vi "Report Driver.vi"(4 "Both XL & PDF":bool, 6 "PDF":bool, 8 "error in":errorcluster, 10 "2D Data":string[][](array[string]), 11 "Header Data":string[](array[string])) -> (0 "error out":errorcluster, 3 "Pathout":path)   [LabVIEW 2017]
uses:
  controls/Excel.ctl
  controls/read.write.ctl
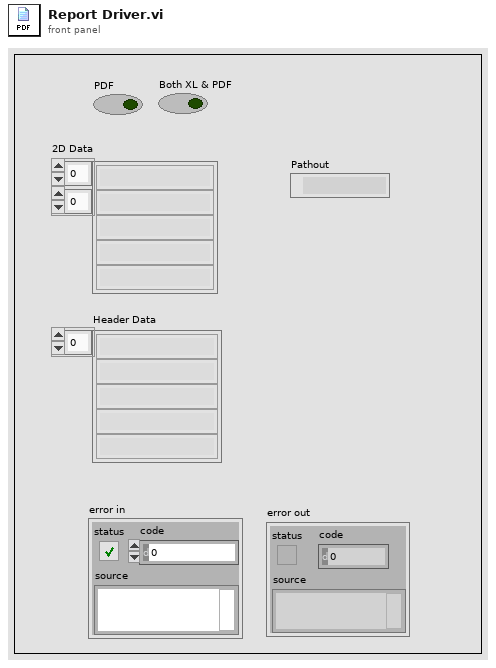
[diagram p1: front panel]
types:
  T1 = typedef "Excel.ctl" = enum16{"Open XL", "Create Hyperlink within Sheet", "Create Hyperlink between Sheets", "Hyperlink Folders", "Read Sheet names", "Print", "Print Preview", "print", "Open WB", "Copy Sheets", "Copy sheet to sheet", "Add Sheets", "Select Sheet", "Paste CLPBRD", "Read 1 Cell", "Read 2D", "Write 1 Cell", "Write 1 Cell No", "Write 2D String", "Write 2D Double", "Write 1D String", "Write 1D Double", "Merge Cells", "Borders", "Save", "Save As PDF", "Get Last Row Column Number", "Close Sheet", "Delete Sheet", "Close WB", "Close XL"}
  T2 = typedef "read.write.ctl" = cluster{"Cell Range":string, "Data 2D":string[][], "Select Sheet":string, "1 Data":string, "Data 1D":string[], "Font col":u32, "Bold":bool, "Font Size":i32, "Inside lines":bool}
  T3 = cluster{"Excel WB Path":path, "Read Only?":bool, "Password":string}
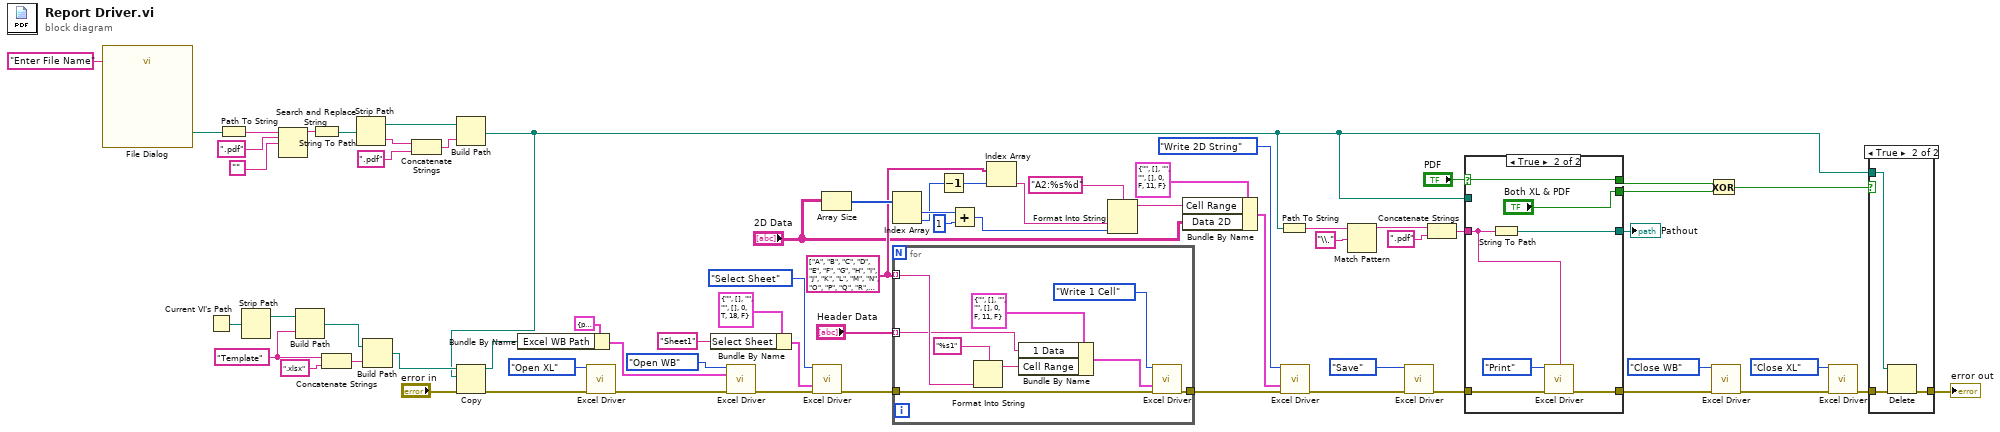
[diagram p0: block diagram]
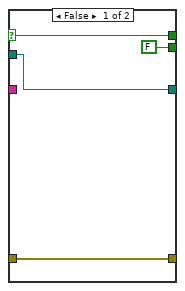
[diagram p3: hidden frame]
diagram:
  w24 = "Template" ("name or relative path")
  w35 = string[] ["A", "B", "C", "D", "E", "F", "G", "H", "I", "J", "K", "L", "M", "N", "O", "P", "Q", "R", "S", "T", "U", "V", "W", "X", "Y", "Z", "AA", "AB", "AC", "AD", "AE", "AF", "AG", "AH", "AI", "AJ", "AK", "AL", "AM", "AN", "AO", "AP", "AQ", "AR", "AS", "AT", "AU", "AV", "AW", "AX", "AY", "AZ", "BA", "BB", "BC", "BD", "BE", "BF", "BG", "BH", "BI", "BJ", "BK", "BL", "BM", "BN", "BO", "BP", "BQ", "BR", "BS", "BT", "BU", "BV", "BW", "BX", "BY", "BZ", "CA", "CB", "CC", "CD", "CE", "CF", "CG", "CH", "CI", "CJ", "CK", "CL", "CM", "CN", "CO", "CP", "CQ", "CR", "CS", "CT", "CU", "CV", "CW", "CX", "CY", "CZ", "DA", "DB", "DC", "DD", "DE", "DF", "DG", "DH", "DI", "DJ", "DK", "DL", "DM", "DN", "DO", "DP", "DQ", "DR", "DS", "DT", "DU", "DV", "DW", "DX", "DY", "DZ", "EA", "EB", "EC", "ED", "EE", "EF", "EG", "EH", "EI", "EJ", "EK", "EL", "EM", "EN", "EO", "EP", "EQ", "ER", "ES", "ET", "EU", "EV", "EW", "EX", "EY", "EZ"] ("array")
  n1 = call "File Dialog"("default name"="Enter File Name") -> ("selected path"=w9:path)  [unwired: 11 in, 3 out]
  n2 = Current VI's Path() -> (path=w20:path)
  n3 = Path To String(path=w9) -> (string=w8:string)
  n4 = Strip Path(path=w20) -> (stripped path=w19:path)  [unwired: 1 out]
  n5 = Search and Replace String(input string=w8, search string=".pdf", replace string="") -> (result string=w5:string)  [unwired: 5 in, 3 out]
  n6 = Build Path(base path=w19, name or relative path=w24) -> (appended path=w25:path)
  n7 = String To Path(string=w5) -> (path=w4:path)
  n8 = Concatenate Strings(w24, ".xlsx" ("string")) -> (w22:string)
  n9 = Strip Path(path=w4) -> (stripped path=w3:path, name=w11:string)
  n10 = Build Path(base path=w25, name or relative path=w22) -> (appended path=w21:path)
  n11 = Concatenate Strings(w11, ".pdf" ("string")) -> (w2:string)
  n12 = Build Path(base path=w3, name or relative path=w2) -> (appended path=w1:path)
  n13 = Copy(8:"error in", 10:w1, 11:w21) -> (0:w28:errorcluster, 3:w30:path)  [unwired: 2 in, 1 out]
  n14 = Bundle By Name(cluster=T3 {"Excel WB Path"=path "", "Read Only?"=FALSE, "Password"=""} ("Workbook"), "Excel WB Path"=w30) -> (w66:T3)
  n15 = call "Excel Driver.vi"("Option"=Excel."Open XL", "error in"=w28) -> ("error out"=w65:errorcluster)  [unwired: 6 in, 7 out]
  n16 = Bundle By Name(cluster=T2 {"Cell Range"="", "Data 2D"=[], "Select Sheet"="", "1 Data"="", "Data 1D"=[], "Font col"=0, "Bold"=TRUE, "Font Size"=18, "Inside lines"=FALSE} ("Write/Read Cell"), "Select Sheet"="Sheet1") -> (w61:T2)
  n17 = call "Excel Driver.vi"("Option"=Excel."Open WB", "Workbook"=w66, "error in"=w65) -> ("error out"=w29:errorcluster)  [unwired: 5 in, 7 out]
  n18 = call "Excel Driver.vi"("Option"=Excel."Select Sheet", "Write/Read Cell"=w61, "error in"=w29) -> ("error out"=w59:errorcluster)  [unwired: 5 in, 7 out]
  n19 = Array Size(array="2D Data") -> (size(s)=w42:i32[])
  n20 = Index Array(array=w42) -> (element #1=w41:i32, element #2=w37:i32)  [unwired: 2 in]
  n21 = for {
    tunnel: w59 -> [w74]
    tunnel: w35 -> [w71] mode=indexing
    tunnel: "Header Data" -> [w70] mode=indexing
    tunnel: [w73] -> w54
    n22 = Format Into String(format string="%s1", w71) -> (resulting string=w69:string)  [unwired: 2 in, 1 out]
    n23 = Bundle By Name(cluster=T2 {"Cell Range"="", "Data 2D"=[], "Select Sheet"="", "1 Data"="", "Data 1D"=[], "Font col"=0, "Bold"=FALSE, "Font Size"=11, "Inside lines"=FALSE} ("Write/Read Cell 2"), "1 Data"=w70, "Cell Range"=w69) -> (w77:T2)
    n24 = call "Excel Driver.vi"("Option"=Excel."Write 1 Cell", "Write/Read Cell"=w77, "error in"=w74) -> ("error out"=w73:errorcluster)  [unwired: 5 in, 7 out]
  }
  n25 = Decrement(x=w37) -> (x-1=w36:i32)
  n26 = Add(x=w41, y=1) -> (x+y=w40:i32)
  n27 = Index Array(array=w35, index=w36) -> (element=w39:string)
  n28 = Format Into String(format string="A2:%s%d", w39, w40) -> (resulting string=w34:string)  [unwired: 2 in, 1 out]
  n29 = Bundle By Name(cluster=T2 {"Cell Range"="", "Data 2D"=[], "Select Sheet"="", "1 Data"="", "Data 1D"=[], "Font col"=0, "Bold"=FALSE, "Font Size"=11, "Inside lines"=FALSE} ("Write/Read Cell 2"), "Cell Range"=w34, "Data 2D"="2D Data") -> (w53:T2)
  n30 = Path To String(path=w1) -> (string=w46:string)
  n31 = call "Excel Driver.vi"("Option"=Excel."Write 2D String", "Write/Read Cell"=w53, "error in"=w54) -> ("error out"=w51:errorcluster)  [unwired: 5 in, 7 out]
  n32 = Match Pattern(string=w46, regular expression="\\.") -> (before substring=w48:string)  [unwired: 1 in, 3 out]
  n33 = call "Excel Driver.vi"("Option"=Excel."Save", "error in"=w51) -> ("error out"=w50:errorcluster)  [unwired: 6 in, 7 out]
  n34 = Concatenate Strings(w48, ".pdf" ("string")) -> (w45:string)
  n35 = case shown="True" "PDF" {
    selector: "PDF" -> [w78 w82]
    tunnel: w50 -> [w81 w85]
    tunnel: w45 -> [_ w87]
    tunnel: [w81 w84] -> w44
    tunnel: [w80 w86] -> w26
    tunnel: w1 -> [w80 _]
    tunnel: [FALSE ("Both XL & PDF") "Both XL & PDF"] -> w15
    tunnel: [w78 w82] -> w13
    frame False {
    }
    frame True {
      n36 = String To Path(string=w87) -> (path=w86:path)
      n37 = call "Excel Driver.vi"("Option"=Excel."Print", "File name"=w87, "error in"=w85) -> ("error out"=w84:errorcluster)  [unwired: 5 in, 7 out]
    }
  }
  "Pathout" <- w26
  n38 = Exclusive Or(1:w15, 2:w13) -> (0:w16:bool)
  n39 = call "Excel Driver.vi"("Option"=Excel."Close WB", "error in"=w44) -> ("error out"=w43:errorcluster)  [unwired: 6 in, 7 out]
  n40 = call "Excel Driver.vi"("Option"=Excel."Close XL", "error in"=w43) -> ("error out"=w18:errorcluster)  [unwired: 6 in, 7 out]
  n41 = case shown="True" w16 {
    tunnel: w18 -> [w89 w92]
    tunnel: [w89 w91] -> w17
    tunnel: w1 -> [_ w90]
    frame False {
    }
    frame True {
      n42 = Delete(path (use dialog)=w90, error in=w92) -> (error out=w91:errorcluster)  [unwired: 3 in, 2 out]
    }
  }
  "error out" <- w17
